vi "BlueLeftAutos.vi"(11 "Auto Array Input":string[][](array[string])) -> (3 "Auto Ran":string)   [LabVIEW 2016]
uses:
  <vilib>/Rock Robotics/Network Tables/NT Read String.vi
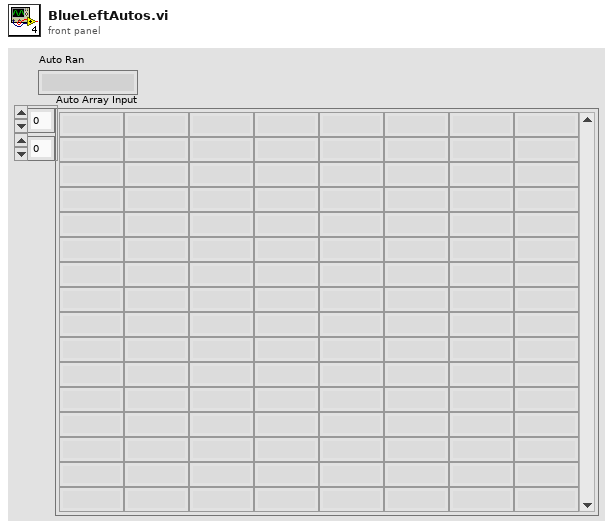
[diagram p1: front panel]
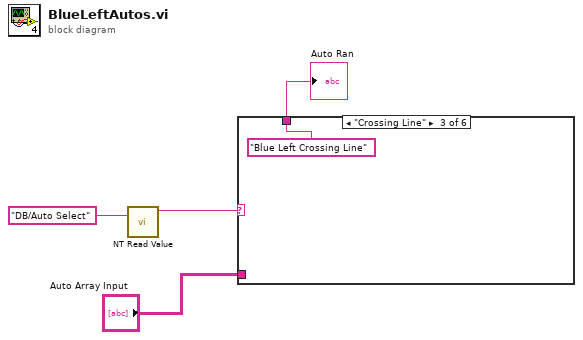
[diagram p0: block diagram]
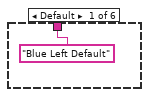
[diagram p2: hidden frame]
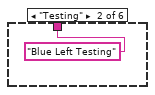
[diagram p3: hidden frame]
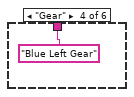
[diagram p4: hidden frame]
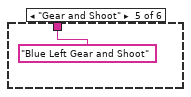
[diagram p5: hidden frame]
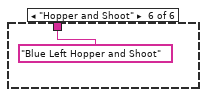
[diagram p6: hidden frame]
diagram:
  n1 = call-poly <vilib>:"NT Read Value.vi"("Name"="DB/Auto Select") -> ("String"=w3:string)  [unwired: 9 in, 1 out]
  n2 = case shown="\"Crossing Line\"" w3 {
    tunnel: ["Blue Left Default" "Blue Left Testing" "Blue Left Crossing Line" "Blue Left Gear" "Blue Left Gear and Shoot" "Blue Left Hopper and Shoot"] -> w2
    tunnel: "Auto Array Input" -> [_ _ _ _ _ _]
    frame Default {
    }
    frame "Testing" {
    }
    frame "Crossing Line" {
    }
    frame "Gear" {
    }
    frame "Gear and Shoot" {
    }
    frame "Hopper and Shoot" {
    }
  }
  "Auto Ran" <- w2
